vi "AddChildtoNode.vi"(8 "error in":errorcluster, 10 "child in":T1, 11 "NISE_CEF_Node in":refnum<class "NISE_CEF_Node.lvclass">) -> (0 "error out":errorcluster, 3 "NISE_CEF_Node out":refnum<class "NISE_CEF_Node.lvclass">)   [LabVIEW 2013, in "NISE_CEF_Node.lvclass"]
uses:
  NISE_CEF_Node.lvclass
  NodeRef.ctl
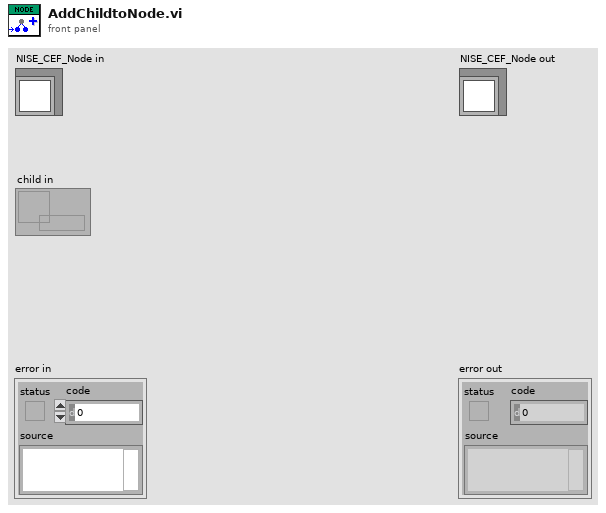
[diagram p1: front panel]
types:
  T1 = typedef "NISE_CEF_Node.lvclass/NodeRef.ctl" = refnum<data-value>
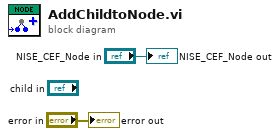
[diagram p0: block diagram]
diagram:
  "error out" <- "error in"
  "NISE_CEF_Node out" <- "NISE_CEF_Node in"
